vi "GPS_2 Port 1 w Compass.vi"() -> ()   [LabVIEW 2009]
uses:
  <vilib>/LabVIEW Targets/FPGA/cRIO/shared/nicrio_ModuleControls/nicrio_cRIO-9871_FlowControlEnum.ctl
  <vilib>/LabVIEW Targets/FPGA/cRIO/shared/nicrio_ModuleControls/nicrio_cRIO-9871_ParityEnum.ctl
  <vilib>/LabVIEW Targets/FPGA/cRIO/shared/nicrio_ModuleControls/nicrio_cRIO-9871_StopBitsEnum.ctl
  <vilib>/LabVIEW Targets/FPGA/cRIO/shared/nicrio_ModuleControls/nicrio_cRIO-9871_DataBitsEnum.ctl
  <vilib>/LabVIEW Targets/FPGA/cRIO/shared/nicrio_ModuleControls/nicrio_cRIO-9871_BaudRateEnum.ctl
  <vilib>/eio/EIOPropertyNode/EIOPropertyNode.xnode
  <vilib>/rvi/eio/nirviEIOPropertyImplementation/nirviEIOPropertyImplementation.xnode
  <vilib>/rvi/eio/common/nirviEmuTemplatePropertySet_errors.vi
  <vilib>/rvi/eio/common/nirviEmuTemplatePropertyGet_errors.vi
  <vilib>/eio/EIOMethodNode/EIOMethodNode.xnode
  <vilib>/rvi/eio/nirviEIOMethodImplementation/nirviEIOMethodImplementation.xnode
  <vilib>/rvi/eio/common/nirviEmuTemplateMethod_errors.vi
  <vilib>/rvi/eio/common/nirviEmuClasses.ctl
panel:
  out "error out":errorcluster
  out "Compass Period (ms)":u16
  in  "Compass Tick Count(mSec)":u16
  in  "Compass Timeout (ms)":i32=150
  out "Compass error out":errorcluster
  out "pitch buffer":u8[](array[numeric])
  out "heading data":u8[](array[numeric])
  out "heading buffer":u8[](array[numeric])
  out "roll data":u8[](array[numeric])
  out "roll buffer":u8[](array[numeric])
  out "pitch data":u8[](array[numeric])
  out "Compass read count":i32
  out "Compass comma count":i32
  out "Compass Heartbeat":bool
  out "Bytes at Port?":bool
  out "New GPS Data":bool
  out "GPS Data":u8[](array[numeric])
  out "Current Buffer":u8[](array[numeric])
  in  "GPS Read Timeout (us)":i32
  # "24"
  # "47"
  # "50"
  # "47"
  # "47"
  # "41"
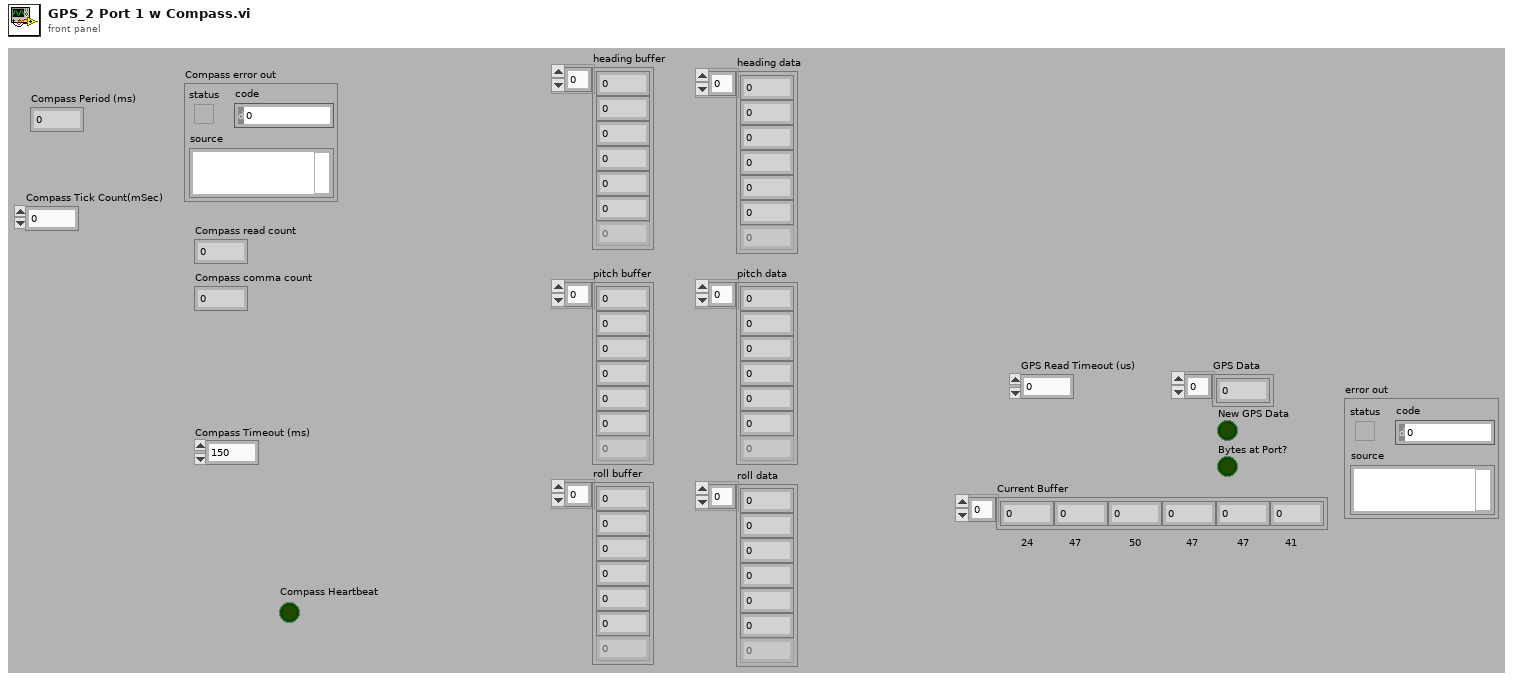
[diagram p1: front panel]
types:
  T1 = typedef "nicrio_cRIO-9871_FlowControlEnum.ctl" = enum8{"None", "Software (XON / XOFF)", "Hardware (RTS / CTS)"}
  T2 = typedef "nicrio_cRIO-9871_ParityEnum.ctl" = enum8{"None", "Odd", "Even", "Mark", "Space"}
  T3 = typedef "nicrio_cRIO-9871_StopBitsEnum.ctl" = enum8{"1", "1.5", "2"}
  T4 = typedef "nicrio_cRIO-9871_DataBitsEnum.ctl" = enum8{"5", "6", "7", "8"}
  T5 = typedef "nicrio_cRIO-9871_BaudRateEnum.ctl" = enum16{"75 bps", "110 bps", "134 bps", "150 bps", "300 bps", "600 bps", "1200 bps", "1800 bps", "2400 bps", "4800 bps", "7200 bps", "9600 bps", "14.4 kbps", "19.2 kbps", "28.8 kbps", "38.4 kbps", "57.6 kbps", "115.2 kbps", "230.4 kbps", "460.8 kbps", "921.6 kbps"}
  T6 = enum16{"Search for LF", "Read heading", "Read pitch", "Read roll"}
  T7 = typedef "nirviEmuClasses.ctl" = enum16{"IO Read", "IO Write", "Method", "Property Read", "Property Write"}
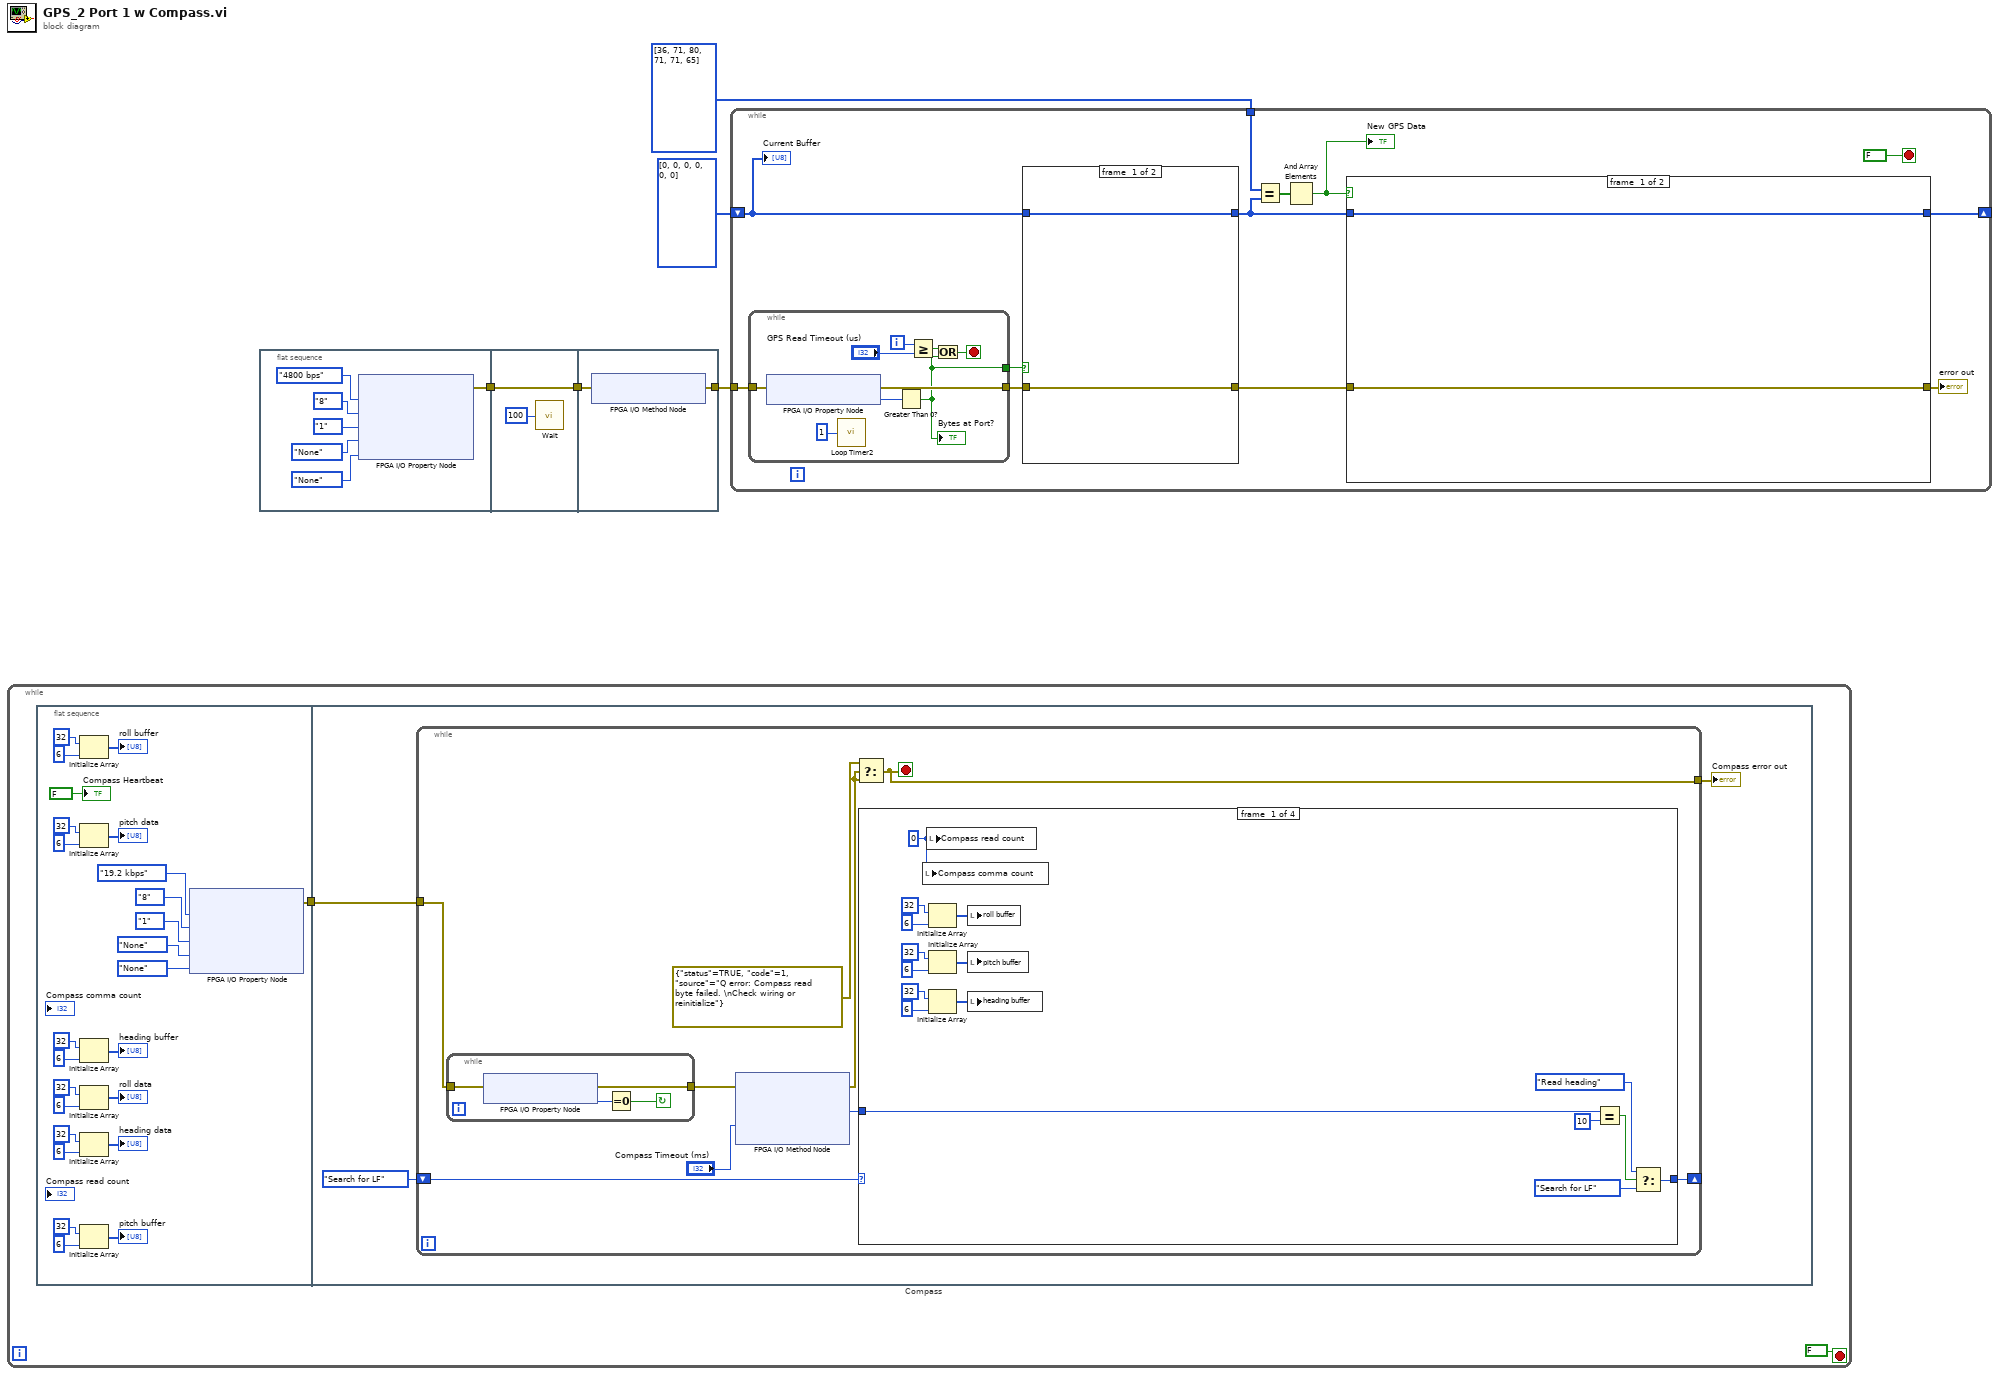
[diagram p0: block diagram]
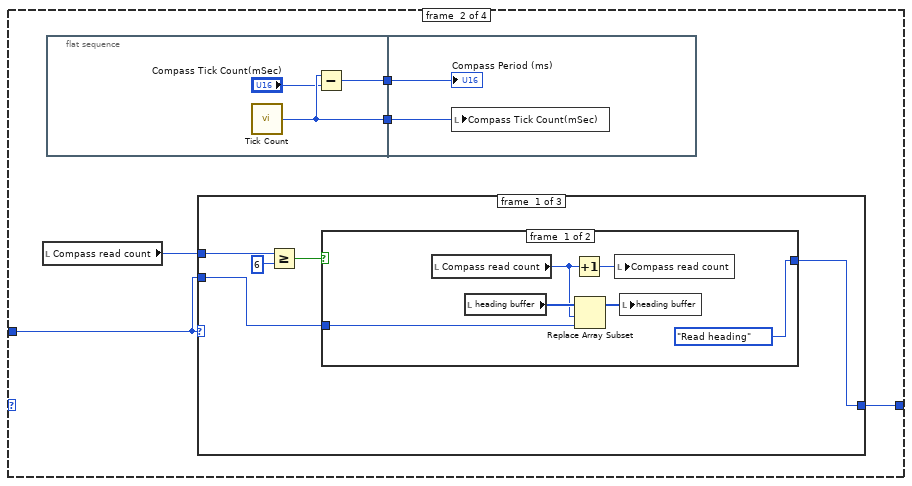
[diagram p2: hidden frame]
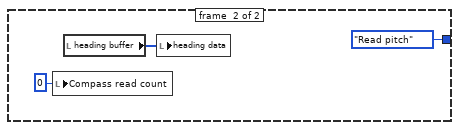
[diagram p3: hidden frame]
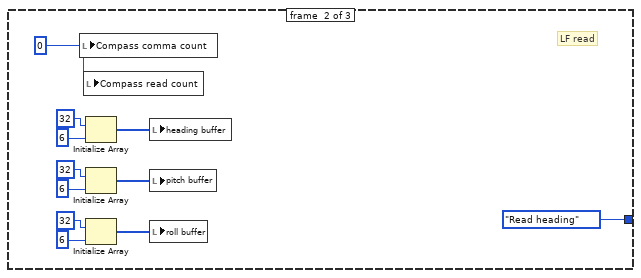
[diagram p4: hidden frame]
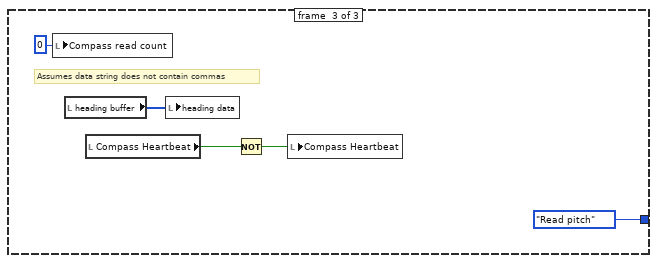
[diagram p5: hidden frame]
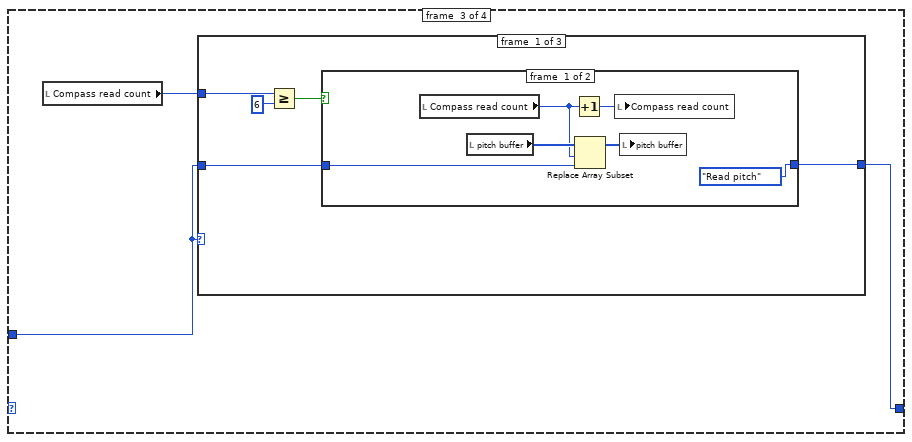
[diagram p6: hidden frame]
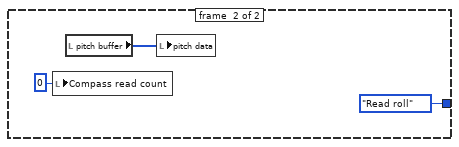
[diagram p7: hidden frame]
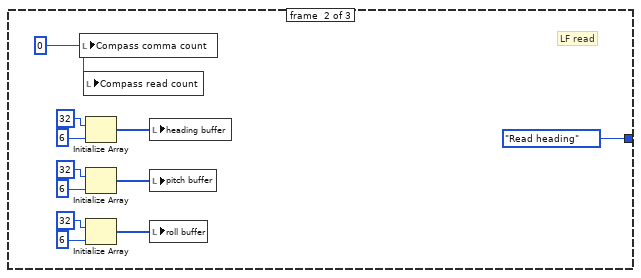
[diagram p8: hidden frame]
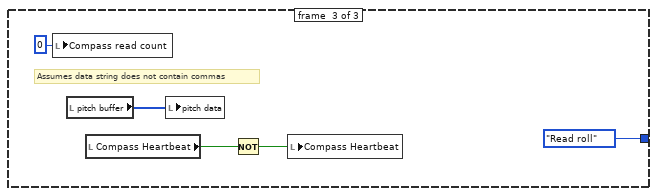
[diagram p9: hidden frame]
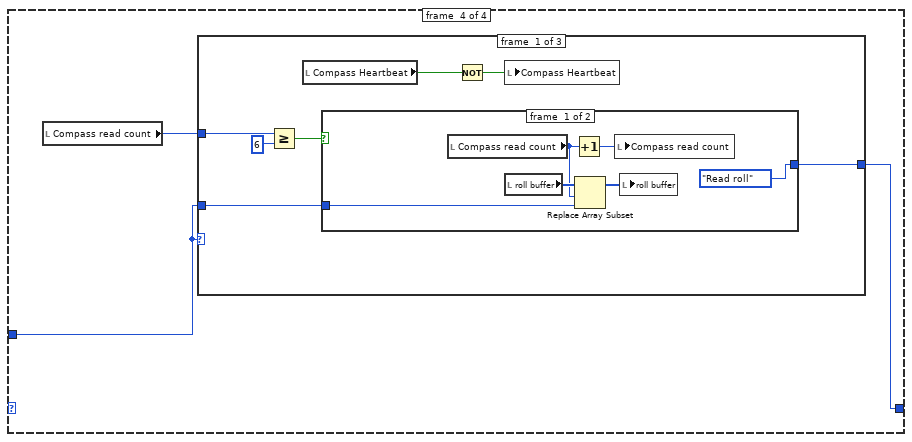
[diagram p10: hidden frame]
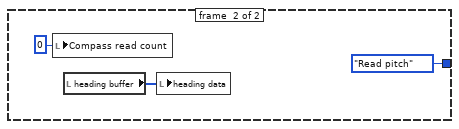
[diagram p11: hidden frame]
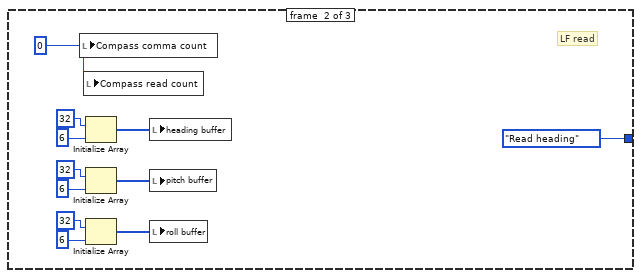
[diagram p12: hidden frame]
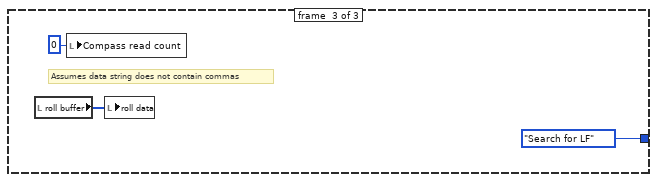
[diagram p13: hidden frame]
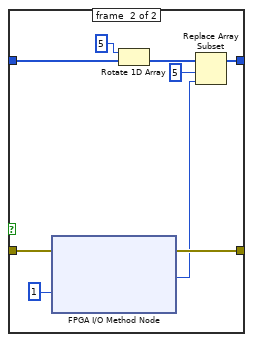
[diagram p14: hidden frame]
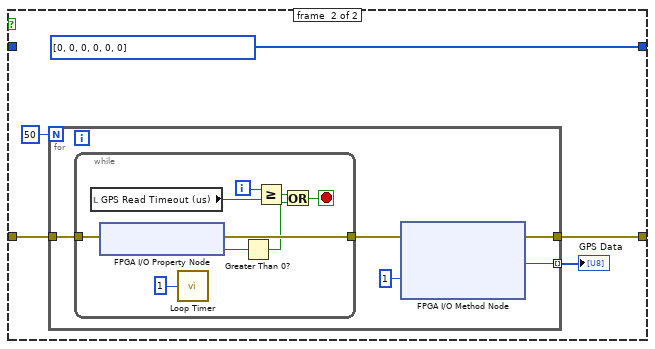
[diagram p15: hidden frame]
diagram:
  n1 = while {
    stop <- FALSE stop-if-true
    n2 = flat-sequence "Compass" {
      tunnel: [w14] -> w7
      tunnel: w7 -> [w81]
      frame #0 {
        n3 = Initialize Array(u8 32 ("y"), 6 ("dimension size")) -> (→"roll buffer":u8[])
        n4 = Initialize Array(u8 32 ("y"), 6 ("dimension size")) -> (→"pitch data":u8[])
        n5 = Initialize Array(u8 32 ("y"), 6 ("dimension size")) -> (→"heading buffer":u8[])
        n6 = Initialize Array(u8 32 ("y"), 6 ("dimension size")) -> (→"roll data":u8[])
        n7 = Initialize Array(u8 32 ("y"), 6 ("dimension size")) -> (→"heading data":u8[])
        n8 = Initialize Array(u8 32 ("y"), 6 ("dimension size")) -> (→"pitch buffer":u8[])
        n9 = xnode "FPGA I/O Property Node"("Baud Rate"=nicrio_cRIO-9871_BaudRateEnum."19.2 kbps", "Data Bits"=nicrio_cRIO-9871_DataBitsEnum."8", "Stop Bits"=nicrio_cRIO-9871_StopBitsEnum."1", "Parity"=nicrio_cRIO-9871_ParityEnum."None", "Flow Control"=nicrio_cRIO-9871_FlowControlEnum."None") -> ("error out"=w14:errorcluster)  [unwired: 2 in, 1 out]
        "Compass Heartbeat" <- FALSE ("SICK Heartbeat")
      }
      frame #1 {
        n10 = while {
          shift-right: [w86] -> _
          shift-left: T6."Search for LF" ("Main states") -> [w87]
          tunnel: [w83] -> w80
          tunnel: w81 -> [w82]
          stop <- w83 stop-if-true
          n11 = while {
            tunnel: [w130] -> w90
            tunnel: w82 -> [w128]
            stop <- w131 continue-if-true
            n12 = xnode "FPGA I/O Property Node"("error in"=w128) -> ("error out"=w130:errorcluster, "Bytes at Port"=w129:u8)  [unwired: 1 in, 1 out]
            n13 = Equal To 0?(x=w129) -> (x = 0?=w131:bool)
          }
          n14 = xnode "FPGA I/O Method Node"("error in"=w90, "Timeout (ms)"="Compass Timeout (ms)") -> ("error out"=w84:errorcluster, "Data"=w88:u8)  [unwired: 1 in, 2 out]
          n15 = Select(t=errorcluster {"status"=TRUE, "code"=1, "source"="Q error: Compass read byte failed. \nCheck wiring or reinitialize"} ("error out"), s=w84, f=w84) -> (s? t:f=w83:errorcluster)
          n16 = case shown="\"Search for LF\", Default" w87 {
            tunnel: w88 -> [w166 w170 w208 w241]
            tunnel: [w163 w171 w209 w242] -> w86
            frame #0 {
              w156 = 0
              n17 = local write "Compass comma count"(w156) -> ()
              n18 = local write "Compass read count"(w156) -> ()
              n19 = Initialize Array(u8 32 ("y"), 6 ("dimension size")) -> (w155:u8[])
              n20 = Initialize Array(u8 32 ("y"), 6 ("dimension size")) -> (w158:u8[])
              n21 = Initialize Array(u8 32 ("y"), 6 ("dimension size")) -> (w157:u8[])
              n22 = local write "roll buffer"(w155) -> ()
              n23 = local write "pitch buffer"(w158) -> ()
              n24 = local write "heading buffer"(w157) -> ()
              n25 = Equal?(x=w166, y=u8 10) -> (x = y?=w164:bool)
              n26 = Select(t=T6."Read heading" ("Main states"), s=w164, f=T6."Search for LF" ("Main states")) -> (s? t:f=w163:T6)
            }
            frame #1 {
              n27 = local read "Compass read count"() -> (w169:i32)
              n28 = flat-sequence {
                tunnel: [w174] -> w168
                tunnel: [w172] -> w167
                tunnel: w168 -> [w176]
                tunnel: w167 -> [w175]
                frame #0 {
                  n29 = call "Tick Count"() -> ("Tick Count(mSec)"=w174:u16)
                  n30 = Subtract(x=w174, y="Compass Tick Count(mSec)") -> (x-y=w172:u16)
                }
                frame #1 {
                  n31 = local write "Compass Tick Count(mSec)"(w176) -> ()
                  "Compass Period (ms)" <- w175
                }
              }
              n32 = case shown="0, Default" w170 {
                tunnel: [w180 T6."Read heading" ("Main states") T6."Read pitch" ("Main states")] -> w171
                tunnel: w170 -> [w181 _ _]
                tunnel: w169 -> [w179 _ _]
                frame #0 {
                  n33 = Greater Or Equal?(x=w179, y=6) -> (x >= y?=w177:bool)
                  n34 = case shown="True" w177 {
                    tunnel: w181 -> [w183 _]
                    tunnel: [T6."Read heading" ("Main states") T6."Read pitch" ("Main states")] -> w180
                    frame #0 {
                      n35 = local read "Compass read count"() -> (w185:i32)
                      n36 = local read "heading buffer"() -> (w186:u8[])
                      n37 = Increment(x=w185) -> (x+1=w187:i32)
                      n38 = Replace Array Subset(array=w186, new element=w183, index=w185) -> (w184:u8[])
                      n39 = local write "Compass read count"(w187) -> ()
                      n40 = local write "heading buffer"(w184) -> ()
                    }
                    frame #1 {
                      n41 = local write "Compass read count"(0 ("Read count")) -> ()
                      n42 = local read "heading buffer"() -> (w190:u8[])
                      n43 = local write "heading data"(w190) -> ()
                    }
                  }
                }
                frame #1 {
                  w198 = 0 ("Comma count")
                  # "LF read"
                  n44 = local write "Compass comma count"(w198) -> ()
                  n45 = local write "Compass read count"(w198) -> ()
                  n46 = Initialize Array(u8 32 ("y"), 6 ("dimension size")) -> (w199:u8[])
                  n47 = Initialize Array(u8 32 ("y"), 6 ("dimension size")) -> (w193:u8[])
                  n48 = Initialize Array(u8 32 ("y"), 6 ("dimension size")) -> (w192:u8[])
                  n49 = local write "heading buffer"(w199) -> ()
                  n50 = local write "pitch buffer"(w193) -> ()
                  n51 = local write "roll buffer"(w192) -> ()
                }
                frame #2 {
                  # "Assumes data string does not contain commas"
                  n52 = local write "Compass read count"(0 ("Comma count")) -> ()
                  n53 = local read "heading buffer"() -> (w206:u8[])
                  n54 = local read "Compass Heartbeat"() -> (w203:bool)
                  n55 = local write "heading data"(w206) -> ()
                  n56 = Not(x=w203) -> (.not. x?=w202:bool)
                  n57 = local write "Compass Heartbeat"(w202) -> ()
                }
              }
            }
            frame #2 {
              n58 = local read "Compass read count"() -> (w207:i32)
              n59 = case shown="0, Default" w208 {
                tunnel: [w213 T6."Read heading" ("Main states") T6."Read roll" ("Main states")] -> w209
                tunnel: w208 -> [w214 _ _]
                tunnel: w207 -> [w212 _ _]
                frame #0 {
                  n60 = Greater Or Equal?(x=w212, y=6) -> (x >= y?=w210:bool)
                  n61 = case shown="False" w210 {
                    tunnel: w214 -> [w216 _]
                    tunnel: [T6."Read pitch" ("Main states") T6."Read roll" ("Main states")] -> w213
                    frame #0 {
                      n62 = local read "Compass read count"() -> (w218:i32)
                      n63 = local read "pitch buffer"() -> (w219:u8[])
                      n64 = Increment(x=w218) -> (x+1=w220:i32)
                      n65 = Replace Array Subset(array=w219, new element=w216, index=w218) -> (w217:u8[])
                      n66 = local write "Compass read count"(w220) -> ()
                      n67 = local write "pitch buffer"(w217) -> ()
                    }
                    frame #1 {
                      n68 = local write "Compass read count"(0 ("Read count")) -> ()
                      n69 = local read "pitch buffer"() -> (w223:u8[])
                      n70 = local write "pitch data"(w223) -> ()
                    }
                  }
                }
                frame #1 {
                  w231 = 0 ("Comma count")
                  # "LF read"
                  n71 = local write "Compass comma count"(w231) -> ()
                  n72 = local write "Compass read count"(w231) -> ()
                  n73 = Initialize Array(u8 32 ("y"), 6 ("dimension size")) -> (w232:u8[])
                  n74 = Initialize Array(u8 32 ("y"), 6 ("dimension size")) -> (w226:u8[])
                  n75 = Initialize Array(u8 32 ("y"), 6 ("dimension size")) -> (w225:u8[])
                  n76 = local write "heading buffer"(w232) -> ()
                  n77 = local write "pitch buffer"(w226) -> ()
                  n78 = local write "roll buffer"(w225) -> ()
                }
                frame #2 {
                  # "Assumes data string does not contain commas"
                  n79 = local write "Compass read count"(0 ("Comma count")) -> ()
                  n80 = local read "pitch buffer"() -> (w239:u8[])
                  n81 = local read "Compass Heartbeat"() -> (w236:bool)
                  n82 = local write "pitch data"(w239) -> ()
                  n83 = Not(x=w236) -> (.not. x?=w235:bool)
                  n84 = local write "Compass Heartbeat"(w235) -> ()
                }
              }
            }
            frame #3 {
              n85 = local read "Compass read count"() -> (w240:i32)
              n86 = case shown="0, Default" w241 {
                tunnel: [w248 T6."Read heading" ("Main states") T6."Search for LF" ("Main states")] -> w242
                tunnel: w241 -> [w249 _ _]
                tunnel: w240 -> [w247 _ _]
                frame #0 {
                  n87 = Greater Or Equal?(x=w247, y=6) -> (x >= y?=w245:bool)
                  n88 = local read "Compass Heartbeat"() -> (w244:bool)
                  n89 = case shown="False" w245 {
                    tunnel: w249 -> [w251 _]
                    tunnel: [T6."Read roll" ("Main states") T6."Read pitch" ("Main states")] -> w248
                    frame #0 {
                      n90 = local read "Compass read count"() -> (w253:i32)
                      n91 = local read "roll buffer"() -> (w254:u8[])
                      n92 = Increment(x=w253) -> (x+1=w255:i32)
                      n93 = Replace Array Subset(array=w254, new element=w251, index=w253) -> (w252:u8[])
                      n94 = local write "Compass read count"(w255) -> ()
                      n95 = local write "roll buffer"(w252) -> ()
                    }
                    frame #1 {
                      n96 = local write "Compass read count"(0 ("Read count")) -> ()
                      n97 = local read "heading buffer"() -> (w258:u8[])
                      n98 = local write "heading data"(w258) -> ()
                    }
                  }
                  n99 = Not(x=w244) -> (.not. x?=w243:bool)
                  n100 = local write "Compass Heartbeat"(w243) -> ()
                }
                frame #1 {
                  w266 = 0 ("Comma count")
                  # "LF read"
                  n101 = local write "Compass comma count"(w266) -> ()
                  n102 = local write "Compass read count"(w266) -> ()
                  n103 = Initialize Array(u8 32 ("y"), 6 ("dimension size")) -> (w267:u8[])
                  n104 = Initialize Array(u8 32 ("y"), 6 ("dimension size")) -> (w261:u8[])
                  n105 = Initialize Array(u8 32 ("y"), 6 ("dimension size")) -> (w260:u8[])
                  n106 = local write "heading buffer"(w267) -> ()
                  n107 = local write "pitch buffer"(w261) -> ()
                  n108 = local write "roll buffer"(w260) -> ()
                }
                frame #2 {
                  # "Assumes data string does not contain commas"
                  n109 = local read "roll buffer"() -> (w272:u8[])
                  n110 = local write "Compass read count"(0 ("Comma count")) -> ()
                  n111 = local write "roll data"(w272) -> ()
                }
              }
            }
          }
        }
        "Compass error out" <- w80
      }
    }
  }
  n112 = flat-sequence {
    tunnel: [w273] -> w3
    tunnel: w3 -> [w326]
    tunnel: [w326] -> w2
    tunnel: w2 -> [w328]
    tunnel: [w327] -> w1
    frame #0 {
      n113 = xnode "FPGA I/O Property Node"("Baud Rate"=nicrio_cRIO-9871_BaudRateEnum."4800 bps" ("Baud Rate 4"), "Data Bits"=nicrio_cRIO-9871_DataBitsEnum."8" ("Data Bits 4"), "Stop Bits"=nicrio_cRIO-9871_StopBitsEnum."1" ("Stop Bits 4"), "Parity"=nicrio_cRIO-9871_ParityEnum."None" ("Parity 4"), "Flow Control"=nicrio_cRIO-9871_FlowControlEnum."None" ("Flow Control 4")) -> ("error out"=w273:errorcluster)  [unwired: 2 in, 1 out]
    }
    frame #1 {
      n114 = call "Wait"("Count(mSec)"=u32 100) -> ()  [unwired: 1 out]
    }
    frame #2 {
      n115 = xnode "FPGA I/O Method Node"("error in"=w328) -> ("error out"=w327:errorcluster)  [unwired: 1 in, 1 out]
    }
  }
  n116 = while {
    tunnel: w1 -> [w350]
    shift-right: [w339] -> _
    shift-left: u8[] [0, 0, 0, 0, 0, 0] -> [w344]
    tunnel: u8[] [36, 71, 80, 71, 71, 65] -> [w343]
    stop <- FALSE stop-if-true
    n117 = while {
      tunnel: w350 -> [w478]
      tunnel: [w477] -> w349
      tunnel: [w476] -> w342
      i -> [w483]
      stop <- w482 stop-if-true
      n118 = xnode "FPGA I/O Property Node"("error in"=w478) -> ("error out"=w477:errorcluster, "Bytes at Port"=w480:u8)  [unwired: 1 in, 1 out]
      n119 = call "Loop Timer2"("Count(uSec)"=u32 1) -> ()  [unwired: 1 out]
      n120 = Greater Than 0?(x=w480) -> (x > 0?=w476:bool)
      "Bytes at Port?" <- w476
      n121 = Greater Or Equal?(x=w483, y="GPS Read Timeout (us)") -> (x >= y?=w481:bool)
      n122 = Or(x=w481, y=w476) -> (x .or. y?=w482:bool)
    }
    n123 = case shown="False" w342 {
      tunnel: w349 -> [w352 w361]
      tunnel: [w352 w359] -> w347
      tunnel: w344 -> [w351 w355]
      tunnel: [w351 w356] -> w340
      frame #0 {
      }
      frame #1 {
        n124 = xnode "FPGA I/O Method Node"("error in"=w361, "Timeout (ms)"=1) -> ("error out"=w359:errorcluster, "Data"=w358:u8)  [unwired: 1 in, 2 out]
        n125 = Rotate 1D Array(1:w355, 2:5 ("n")) -> (0:w354:u8[])
        n126 = Replace Array Subset(array=w354, new element=w358, index=5) -> (w356:u8[])
      }
    }
    n127 = Equal?(x=w343, y=w340) -> (x = y?=w348:bool[])
    n128 = And Array Elements(Boolean array=w348) -> (logical AND=w346:bool)
    "New GPS Data" <- w346
    n129 = case shown="True" w346 {
      tunnel: w347 -> [w400 w404]
      tunnel: [w400 w402] -> w341
      tunnel: w340 -> [w399 _]
      tunnel: [w399 u8[] [0, 0, 0, 0, 0, 0]] -> w339
      frame #0 {
      }
      frame #1 {
        n130 = for {
          N: 50 -> [_]
          tunnel: w404 -> [w410]
          tunnel: [w407] -> w403 mode=indexing
          tunnel: [w406] -> w402
          n131 = while {
            tunnel: w410 -> [w414]
            tunnel: [w413] -> w409
            i -> [w418]
            stop <- w417 stop-if-true
            n132 = local read "GPS Read Timeout (us)"() -> (w411:i32)
            n133 = xnode "FPGA I/O Property Node"("error in"=w414) -> ("error out"=w413:errorcluster, "Bytes at Port"=w415:u8)  [unwired: 1 in, 1 out]
            n134 = call "Loop Timer"("Count(uSec)"=u32 1) -> ()  [unwired: 1 out]
            n135 = Greater Than 0?(x=w415) -> (x > 0?=w412:bool)
            n136 = Greater Or Equal?(x=w418, y=w411) -> (x >= y?=w416:bool)
            n137 = Or(x=w416, y=w412) -> (x .or. y?=w417:bool)
          }
          n138 = xnode "FPGA I/O Method Node"("error in"=w409, "Timeout (ms)"=1) -> ("error out"=w406:errorcluster, "Data"=w407:u8)  [unwired: 1 in, 2 out]
        }
        "GPS Data" <- w403
      }
    }
    "error out" <- w341
    "Current Buffer" <- w344
  }
